vi "Find intersection of two straight lines.vi"(8 "Intercept 1":dbl=-3.365107226483396e-10, 9 "Slope 1":dbl=2.99895290773469e-09, 10 "Intercept 0":dbl=1.6090011156861096e-14, 11 "Slope 0":dbl=1.3274900211188954e-09) -> (2 "Y of intersection":dbl=2.6728854291553117e-10, 3 "X of intersection":dbl=0.2013366945531535)   [LabVIEW 2016]
panel:
  out "XY Graph":cluster{dbl[], dbl[]}[](graph)
  in  "X Data points":dbl=4792.0
  in  "Final X":dbl=65.0
  in  "Initial X":dbl=-100.0
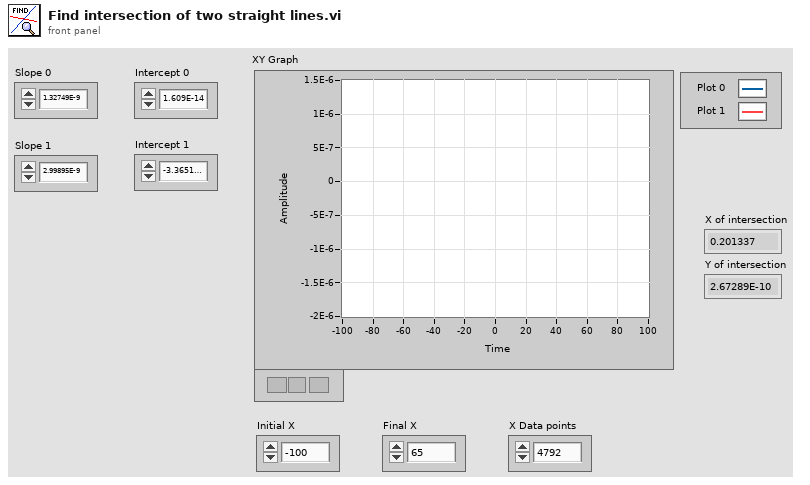
[diagram p1: front panel]
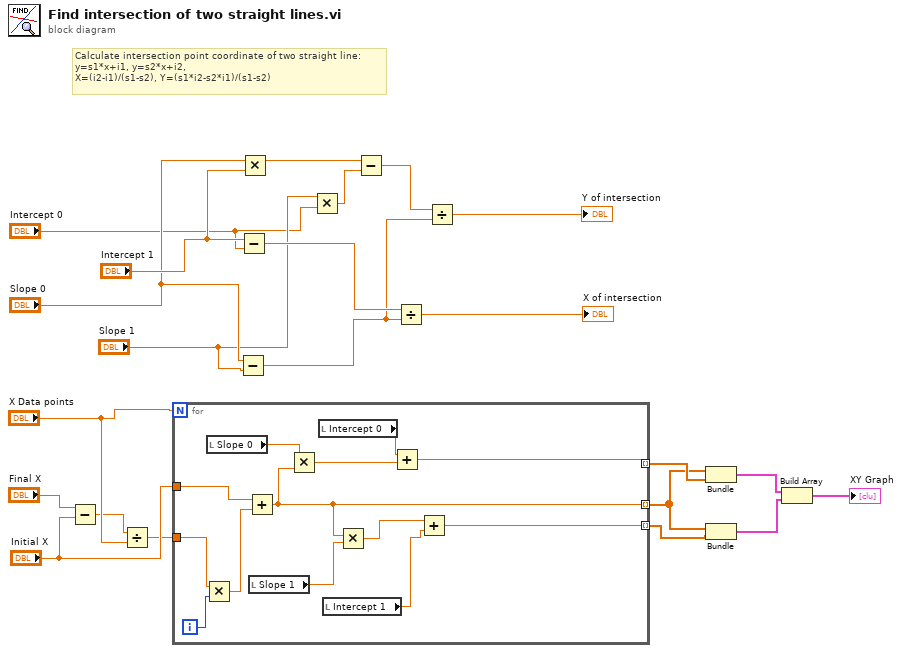
[diagram p0: block diagram]
diagram:
  # "Calculate intersection point coordinate of two straight line:\ny=s1*x+i1, y=s2*x+i2,\nX=(i2-i1)/(s1-s2), Y=(s1*i2-s2*i1)/(s1-s2)"
  n1 = Subtract(x="Final X", y="Initial X") -> (x-y=w9:dbl)
  n2 = Divide(x=w9, y="X Data points") -> (x/y=w7:dbl)
  n3 = for {
    N: "X Data points" -> [_]
    tunnel: "Initial X" -> [w35]
    tunnel: w7 -> [w34]
    tunnel: [w25] -> w5 mode=indexing
    tunnel: [w24] -> w6 mode=indexing
    tunnel: [w23] -> w4 mode=indexing
    i -> [w33]
    n4 = Multiply(x=w34, y=w33) -> (x*y=w32:dbl)
    n5 = local read "Slope 0"() -> (w31:dbl)
    n6 = Add(x=w35, y=w32) -> (x+y=w25:dbl)
    n7 = local read "Slope 1"() -> (w28:dbl)
    n8 = Multiply(x=w31, y=w25) -> (x*y=w30:dbl)
    n9 = local read "Intercept 0"() -> (w29:dbl)
    n10 = local read "Intercept 1"() -> (w26:dbl)
    n11 = Multiply(x=w25, y=w28) -> (x*y=w27:dbl)
    n12 = Add(x=w29, y=w30) -> (x+y=w24:dbl)
    n13 = Add(x=w27, y=w26) -> (x+y=w23:dbl)
  }
  n14 = Subtract(x="Slope 0", y="Slope 1") -> (x-y=w13:dbl)
  n15 = Subtract(x="Intercept 1", y="Intercept 0") -> (x-y=w22:dbl)
  n16 = Multiply(x="Slope 0", y="Intercept 1") -> (x*y=w18:dbl)
  n17 = Multiply(x="Slope 1", y="Intercept 0") -> (x*y=w15:dbl)
  n18 = Subtract(x=w18, y=w15) -> (x-y=w14:dbl)
  n19 = Divide(x=w22, y=w13) -> (x/y=→"X of intersection":dbl)
  n20 = Divide(x=w14, y=w13) -> (x/y=→"Y of intersection":dbl)
  n21 = Bundle(w5, w6) -> (w3:cluster{dbl[], dbl[]})  [unwired: 1 in]
  n22 = Bundle(w5, w4) -> (w2:cluster{dbl[], dbl[]})  [unwired: 1 in]
  n23 = Build Array(w3, w2) -> (→"XY Graph":cluster{dbl[], dbl[]}[])
